vi "Agilent SNA Read Identification.vi"(8 "error in (no error)":errorcluster, 11 "VISA Resource Names":T2) -> (0 "error out":errorcluster, 2 "Instrument Info":T1, 3 "dup VISA Resource Names":T2)   [LabVIEW 2011]
uses:
  TypeDefs/Agilent SNA VISA.ctl
  TypeDefs/Agilent SNA Instrument Info.ctl
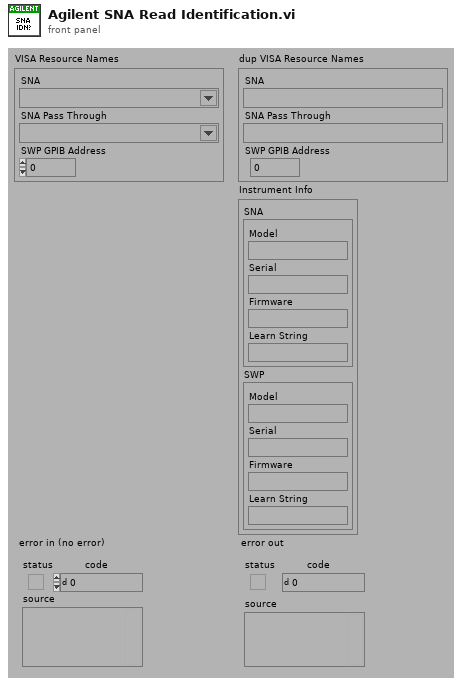
[diagram p1: front panel]
types:
  T1 = typedef "Agilent SNA Instrument Info.ctl" = cluster{"SNA":cluster{"Model":string, "Serial":string, "Firmware":string, "Learn String":string}, "SWP":cluster{"Model":string, "Serial":string, "Firmware":string, "Learn String":string}}
  T2 = typedef "Agilent SNA VISA.ctl" = cluster{"SNA":refnum<visa-resource-name>, "SNA Pass Through":refnum<visa-resource-name>, "SWP GPIB Address":i32}
  T3 = typedef "Agilent SNA Model.ctl" = enum16{"Not Supported", "8757X"}
  T4 = typedef "Agilent SNA SWP Model.ctl" = enum16{"Not Supported", "836XXX", "8375XX", "E82X7D"}
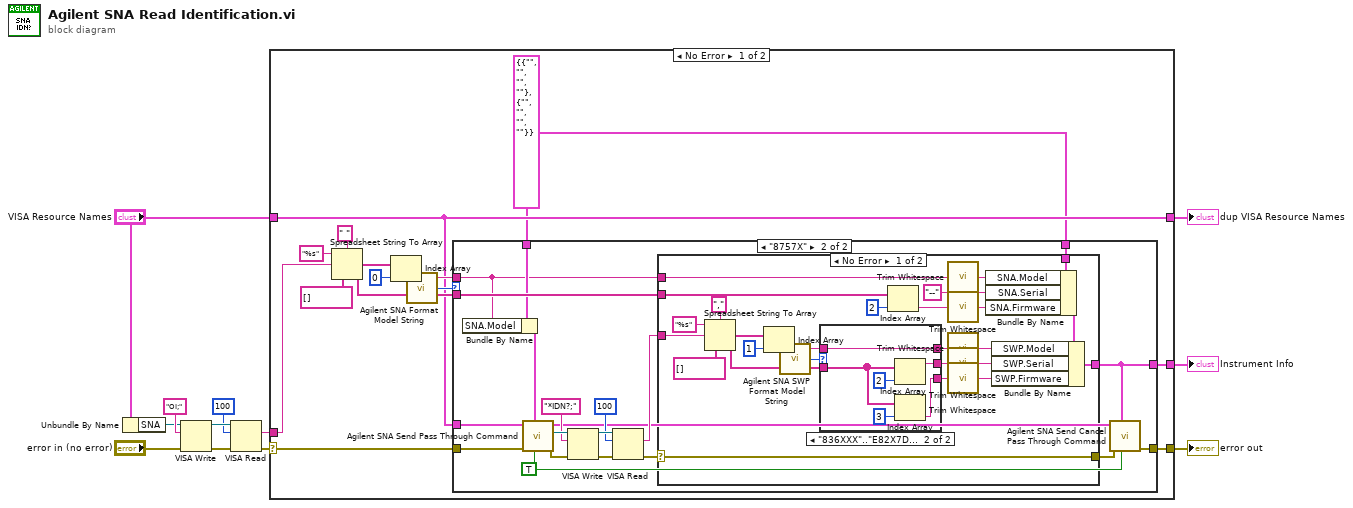
[diagram p0: block diagram]
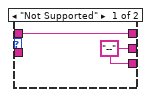
[diagram p3: hidden frame]
diagram:
  n1 = Unbundle By Name("VISA Resource Names") -> ("SNA"=w6:refnum<visa-resource-name>)
  n2 = VISA Write(VISA resource name=w6, write buffer="OI;", error in (no error)="error in (no error)") -> (VISA resource name out=w10:refnum<visa-resource-name>, error out=w8:errorcluster)  [unwired: 1 out]
  n3 = VISA Read(VISA resource name=w10, byte count=u32 100, error in (no error)=w8) -> (read buffer=w12:string, error out=w2:errorcluster)  [unwired: 2 out]
  n4 = case shown="No Error" w2 {
    selector: w2 -> [w15 w84]
    tunnel: w12 -> [w25 _]
    tunnel: [w17 w84] -> w5
    tunnel: [w16 _] -> w4
    tunnel: "VISA Resource Names" -> [w14 w83]
    tunnel: [w14 w83] -> w1
    frame No Error {
      w13 = T1 {"SNA"={"Model"="", "Serial"="", "Firmware"="", "Learn String"=""}, "SWP"={"Model"="", "Serial"="", "Firmware"="", "Learn String"=""}} ("Agilent SNA & SWP")
      n5 = Spreadsheet String To Array(delimiter (Tab)=" ", format string="%s", spreadsheet string=w25, array type (2D Dbl)=string[] []) -> (array=w20:string[])
      n6 = Index Array(array=w20, index=0) -> (element=w18:string)
      n7 = call "Agilent SNA Format Model String.vi"("Model String"=w18) -> ("Model"=w19:T3)
      n8 = case shown="\"8757X\"" w19 {
        tunnel: w20 -> [_ w47]
        tunnel: w18 -> [_ w43]
        tunnel: w15 -> [w27 w46]
        tunnel: [w27 w34] -> w17
        tunnel: [w26 w35] -> w16
        tunnel: w13 -> [w26 w45]
        tunnel: w13 -> [_ w44]
        tunnel: w14 -> [_ w42]
        frame "Not Supported" {
        }
        frame "8757X" {
          w28 = TRUE ("SCPI? (F)")
          n9 = Bundle By Name(cluster=w44, "SNA.Model"=w43) -> (w33:T1)
          n10 = call "Agilent SNA Send Pass Through Command.vi"("SCPI? (F)"=w28, "Agilent SNA & SWP"=w33, "error in (no error)"=w46, "VISA Resource Names"=w42) -> ("error out"=w40:errorcluster, "SNA Pass Through"=w41:refnum<visa-resource-name>, "dup VISA Resource Names"=w30:T2)  [unwired: 5 out]
          n11 = VISA Write(VISA resource name=w41, write buffer="*IDN?;", error in (no error)=w40) -> (VISA resource name out=w39:refnum<visa-resource-name>, error out=w32:errorcluster)  [unwired: 1 out]
          n12 = VISA Read(VISA resource name=w39, byte count=u32 100, error in (no error)=w32) -> (read buffer=w31:string, error out=w29:errorcluster)  [unwired: 2 out]
          n13 = case shown="No Error" w29 {
            selector: w29 -> [w61 w82]
            tunnel: w47 -> [w72 _]
            tunnel: [w70 w81] -> w35
            tunnel: w45 -> [w68 w81]
            tunnel: w43 -> [w59 _]
            tunnel: w31 -> [w64 _]
            tunnel: [w61 w82] -> w36
            frame No Error {
              n14 = Spreadsheet String To Array(delimiter (Tab)=",", format string="%s", spreadsheet string=w64, array type (2D Dbl)=string[] []) -> (array=w62:string[])
              n15 = Index Array(array=w62, index=1) -> (element=w63:string)
              n16 = call "Agilent SNA SWP Format Model String.vi"("Model String"=w63) -> ("Model"=w65:T4)
              n17 = case shown="\"836XXX\"..\"E82X7D\"" w65 {
                tunnel: [w73 w80] -> w57
                tunnel: [w74 w78] -> w56
                tunnel: [w74 w76] -> w55
                tunnel: w63 -> [w73 w80]
                tunnel: w62 -> [_ w75]
                frame "Not Supported" {
                  w74 = "--"
                }
                frame "836XXX".."E82X7D" {
                  n18 = Index Array(array=w75, index=2) -> (element=w78:string)
                  n19 = Index Array(array=w75, index=3) -> (element=w76:string)
                }
              }
              n20 = Index Array(array=w72, index=2) -> (element=w58:string)
              n21 = call <vilib>:"Trim Whitespace.vi"("string"=w59) -> ("trimmed string"=w50:string)  [unwired: 1 in]
              n22 = call <vilib>:"Trim Whitespace.vi"("string"=w58) -> ("trimmed string"=w51:string)  [unwired: 1 in]
              n23 = call <vilib>:"Trim Whitespace.vi"("string"=w57) -> ("trimmed string"=w52:string)  [unwired: 1 in]
              n24 = call <vilib>:"Trim Whitespace.vi"("string"=w56) -> ("trimmed string"=w53:string)  [unwired: 1 in]
              n25 = call <vilib>:"Trim Whitespace.vi"("string"=w55) -> ("trimmed string"=w54:string)  [unwired: 1 in]
              n26 = Bundle By Name(cluster=w68, "SNA.Model"=w50, "SNA.Serial"="--", "SNA.Firmware"=w51) -> (w60:T1)
              n27 = Bundle By Name(cluster=w60, "SWP.Model"=w52, "SWP.Serial"=w53, "SWP.Firmware"=w54) -> (w70:T1)
            }
            frame Error {
            }
          }
          n28 = call "Agilent SNA Send Cancel Pass Through Command.vi"("SCPI? (F)"=w28, "Agilent SNA & SWP"=w35, "error in (no error)"=w36, "VISA Resource Names"=w30) -> ("error out"=w34:errorcluster)  [unwired: 7 out]
        }
      }
    }
    frame Error {
    }
  }
  "error out" <- w5
  "dup VISA Resource Names" <- w1
  "Instrument Info" <- w4
